vi "Vision Shot Info.vi"(10 "fAr dist":dbl, 11 "Distance":dbl) -> (2 "is we far b0ss?":bool)   [LabVIEW 2016]
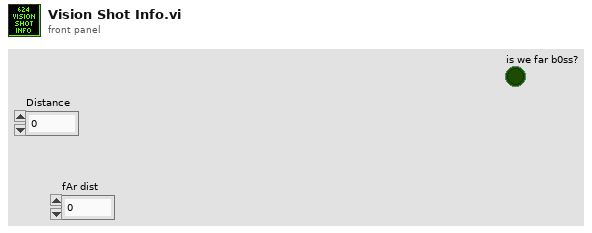
[diagram p1: front panel]
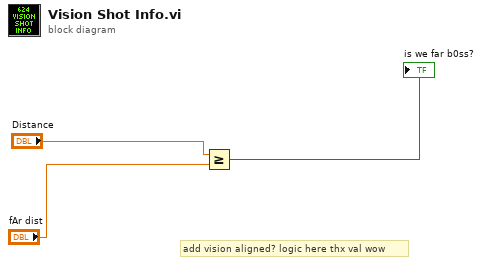
[diagram p0: block diagram]
diagram:
  # "add vision aligned? logic here thx val wow"
  n1 = Greater Or Equal?(x="Distance", y="fAr dist") -> (x >= y?=→"is we far b0ss?":bool)
